vi "LineDetectColorSensor.vi"(11 "NXT In":T1) -> (2 "CrossedLine?":bool, 3 "NXT Out":T1 caption="NXT")   [LabVIEW 2012]
uses:
  <vilib>/NXT/Subs/LVHSConnector.ctl
  <vilib>/NXT/LegoClasses/BrickReference/BrickReference.lvclass
  <vilib>/NXT/HiTechnic/HiTechnic Controls/HiTechnic Port.ctl
  <vilib>/NXT/Block Support/NXT_InputPort.ctl
  <vilib>/NXT/HiTechnic/HiTechnic SubVIs/HiTechnic Color Sensor Active Color.vi
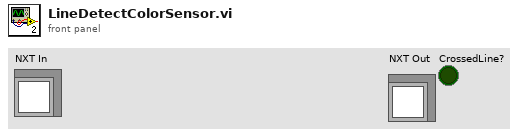
[diagram p1: front panel]
types:
  T1 = typedef "LVHSConnector.ctl" = refnum<class "BrickReference.lvclass">
  T2 = typedef "HiTechnic Port.ctl" = cluster{"Port":T3, "MUX Port":u8}
  T3 = typedef "NXT_InputPort.ctl" = u8
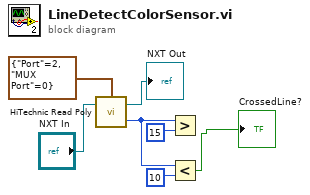
[diagram p0: block diagram]
diagram:
  n1 = call-poly <vilib>:"HiTechnic Read Poly.vi"("NXT"="NXT In", "Port/MUX"=T2 {"Port"=2, "MUX Port"=0}) -> ("Color Number"=w5:i32, "NXT"=→"NXT Out":T1)  [unwired: 1 in]
  n2 = Greater?(x=w5, y=15) -> ()  [unwired: 1 out]
  n3 = Less?(x=w5, y=10) -> (x < y?=→"CrossedLine?":bool)
